vi "Set Command Parameters.vi"(8 "error in (no error)":errorcluster, 10 "Command Parameters In":T1 {"Linkages"."Channel Ref" format="%.0x"}, 11 "Item Ref in":T4 format="%.0x") -> (0 "error out":errorcluster, 2 "Command Parameters Out":T1 {"Linkages"."Channel Ref" format="%.0x"}, 3 "Item Ref out":T4 format="%.0x")   [LabVIEW 2018, in "Instrument Addon Scripting API.lvlib"]
uses:
  Instrument Addon Scripting API.lvlib
  <vilib>/NI Veristand/Custom Device API/Custom Device Item Ref.ctl
  TypeDefs/Command Settings.ctl
  TypeDefs/Padding.ctl
  TypeDefs/Linked Channel.ctl
  Addon/Addon Shared/SubVIs/Constants.vi
  <vilib>/NI Veristand/Custom Device API/Set Item Property (String).vi
  <vilib>/NI Veristand/Custom Device API/Set Item Property (String Array).vi
  <vilib>/NI Veristand/Custom Device API/Set Item Property (Boolean).vi
  <vilib>/NI Veristand/Custom Device API/Set Item Property (U32).vi
  Addon/Addon Shared/Instrument Addon Shared.lvlib
  <vilib>/NI VeriStand/Custom Device API/Custom Device API.lvlib
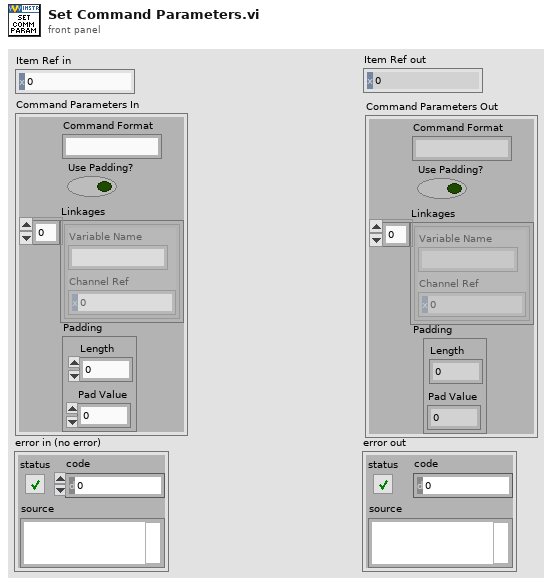
[diagram p1: front panel]
types:
  T1 = typedef "Instrument Addon Scripting API.lvlib/Command Settings.ctl" = cluster{"Command Format":string, "Use Padding?":bool, "Padding":T2, "Linkages":T3}
  T2 = typedef "Instrument Addon Scripting API.lvlib/Padding.ctl" = cluster{"Length":u32, "Pad Value":u8}
  T3 = typedef "Instrument Addon Scripting API.lvlib/Linked Channel.ctl" = cluster{"Channel Ref":T4, "Variable Name":string}[]
  T4 = typedef "Custom Device API.lvlib/Custom Device Item Ref.ctl" = u64
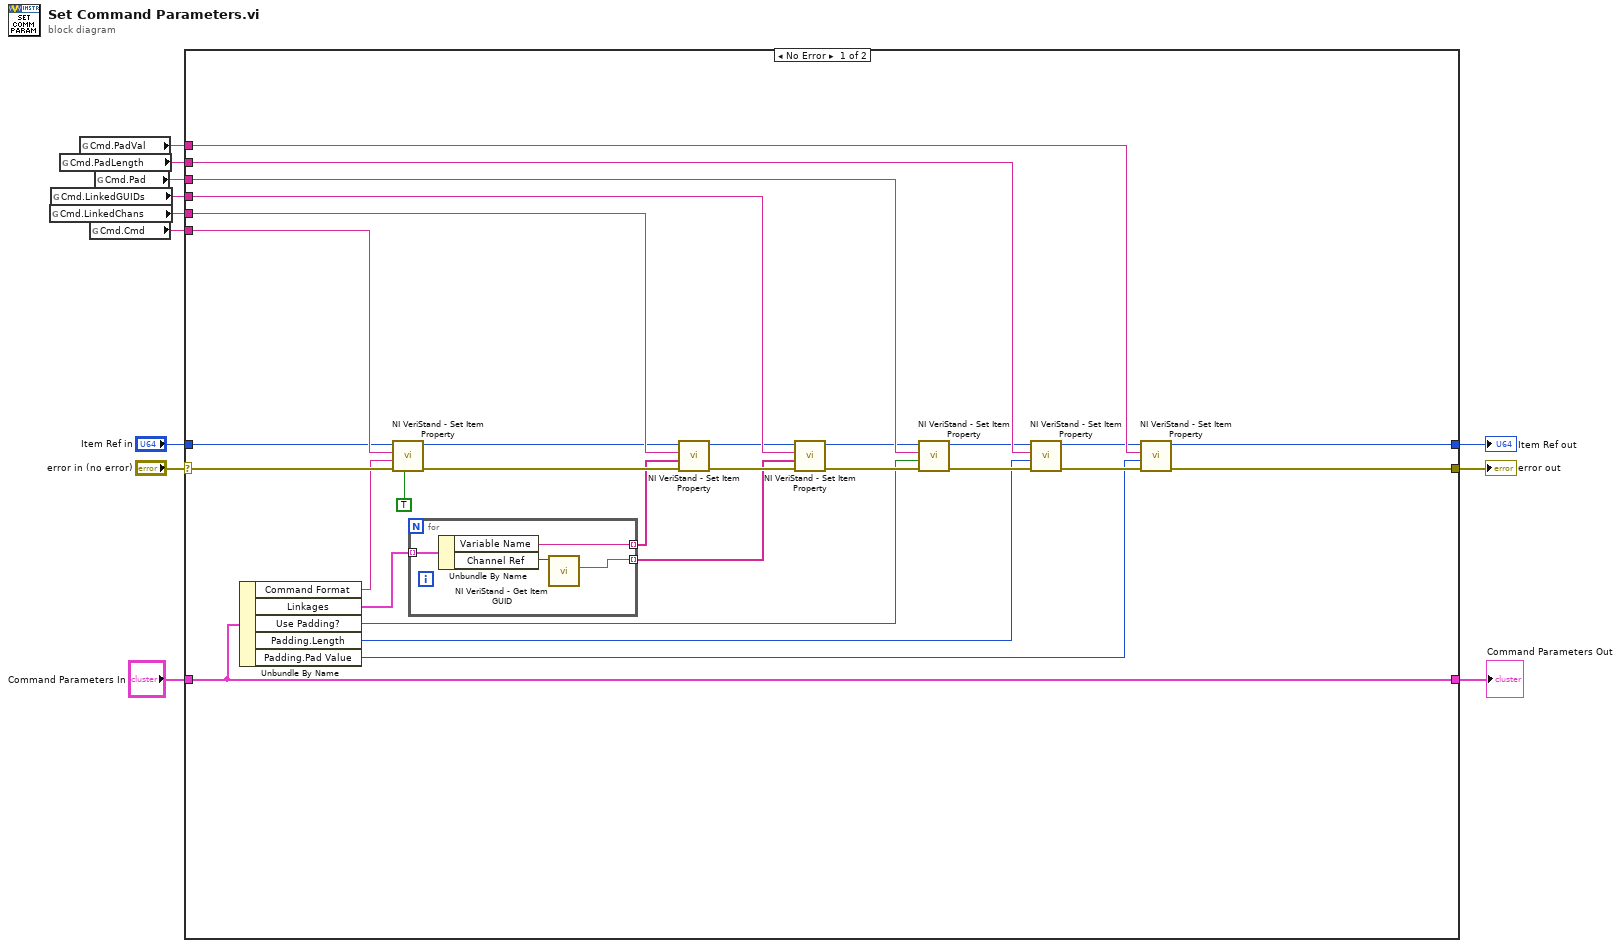
[diagram p0: block diagram]
diagram:
  n1 = global read "Constants.vi" "Cmd.LinkedChans"() -> (w7:string)
  n2 = global read "Constants.vi" "Cmd.LinkedGUIDs"() -> (w6:string)
  n3 = global read "Constants.vi" "Cmd.PadLength"() -> (w4:string)
  n4 = global read "Constants.vi" "Cmd.PadVal"() -> (w3:string)
  n5 = global read "Constants.vi" "Cmd.Cmd"() -> (w8:string)
  n6 = global read "Constants.vi" "Cmd.Pad"() -> (w5:string)
  n7 = case shown="No Error" "error in (no error)" {
    selector: "error in (no error)" -> [w37 w48]
    tunnel: w8 -> [w41 _]
    tunnel: [w40 w46] -> w11
    tunnel: "Item Ref in" -> [w39 w46]
    tunnel: "Command Parameters In" -> [w36 w47]
    tunnel: [w38 w48] -> w10
    tunnel: [w36 w47] -> w1
    tunnel: w7 -> [w35 _]
    tunnel: w6 -> [w34 _]
    tunnel: w5 -> [w33 _]
    tunnel: w4 -> [w32 _]
    tunnel: w3 -> [w31 _]
    frame No Error {
      n8 = Unbundle By Name(w36) -> ("Command Format"=w30:string, "Linkages"=w28:T3, "Use Padding?"=w15:bool, "Padding.Length"=w14:u32, "Padding.Pad Value"=w13:u8)
      n9 = call-poly <vilib>:"NI VeriStand - Set Item Property.vi"("Binary String (T)"=TRUE, "error in (no error)"=w37, "Value"=w30, "Property Name"=w41, "Item Ref in"=w39) -> ("error out"=w26:errorcluster, "Item Ref out"=w27:T4)  [unwired: 4 in, 1 out]
      n10 = for {
        tunnel: w28 -> [w45] mode=indexing
        tunnel: [w44] -> w16 mode=indexing
        tunnel: [w42] -> w17 mode=indexing
        n11 = Unbundle By Name(w45) -> ("Variable Name"=w44:string, "Channel Ref"=w43:T4)
        n12 = call <vilib>:"NI VeriStand - Get Item GUID.vi"("Item Ref in"=w43) -> ("GUID"=w42:string)  [unwired: 8 in, 2 out]
      }
      n13 = call-poly <vilib>:"NI VeriStand - Set Item Property.vi"("error in (no error)"=w26, "Value"=w16, "Property Name"=w35, "Item Ref in"=w27) -> ("error out"=w25:errorcluster, "Item Ref out"=w18:T4)  [unwired: 5 in, 1 out]
      n14 = call-poly <vilib>:"NI VeriStand - Set Item Property.vi"("error in (no error)"=w25, "Value"=w17, "Property Name"=w34, "Item Ref in"=w18) -> ("error out"=w24:errorcluster, "Item Ref out"=w19:T4)  [unwired: 5 in, 1 out]
      n15 = call-poly <vilib>:"NI VeriStand - Set Item Property.vi"("error in (no error)"=w24, "Value"=w15, "Property Name"=w33, "Item Ref in"=w19) -> ("error out"=w23:errorcluster, "Item Ref out"=w20:T4)  [unwired: 5 in, 1 out]
      n16 = call-poly <vilib>:"NI VeriStand - Set Item Property.vi"("error in (no error)"=w23, "Value"=w14, "Property Name"=w32, "Item Ref in"=w20) -> ("error out"=w22:errorcluster, "Item Ref out"=w21:T4)  [unwired: 5 in, 1 out]
      n17 = call-poly <vilib>:"NI VeriStand - Set Item Property.vi"("error in (no error)"=w22, "Value"=w13, "Property Name"=w31, "Item Ref in"=w21) -> ("error out"=w38:errorcluster, "Item Ref out"=w40:T4)  [unwired: 5 in, 1 out]
    }
    frame Error {
    }
  }
  "error out" <- w10
  "Item Ref out" <- w11
  "Command Parameters Out" <- w1
